vi "weight_experimental6.vi"(7 "Stop read":bool, 9 "weight source":bool, 10 "Tick":u32=100, 11 "PV weight":dbl caption="g" format="%#.0f") -> (0 "Vibration":bool caption="Вибрация", 1 "Q 2":dbl caption="mg/s" format="%#.0f", 2 "Q 1":dbl caption="mg/s" format="%#.0f", 3 "Weight 1":dbl caption="g" format="%#.0f", 5 "This VI":refnum<vi>)   [LabVIEW 2019]
uses:
  <vilib>/Analysis/baseanly.llb/Mean (DBL).vi
  Logik/fronts.vi
  Trigers/RS.vi
  Timer Delay/Timers.lvlib
  <vilib>/Analysis/NI_AALBase.lvlib
  Userlib.lvlib
  <vilib>/ptbypt/NI_PtbyPt.lvlib
panel:
  in  "Tab Control":T1(tab)=enum."Настр Ohaos"
  out "dM 2":dbl caption="g" format="%#.0f"
  out "dM 1":dbl caption="g" format="%#.0f"
  in  "Tare":dbl caption="g" format="%#.0f"
  in  "<0>":bool
  in  "<вес>":bool
  in  "k":dbl=1.0 caption="g" format="%#.3f"
  in  "Вес":dbl caption="g" format="%#.0f"
  in  "Период оценки скорости, с":i32=30
  in  "Период оценки вибрации, с":i32=20
  in  "Период усреднения, с":i32=150
  in  "Вырезать после сработки, с":i32=12
  in  "порог":dbl=480.0
  in  "Период усреднения 2":i32=50
  in  "Период оценки скорости OHAOS, с":i32=15
  in  "Период оценки вибрации OHAOS, с":i32=10
  in  "Период усреднения OHAOS, с":i32=120
  in  "Вырезать после сработки OHAOS, с":i32=5
  in  "порог OHAOS":dbl=240.0
  in  "Период усреднения OHAOS 2":i32=30
  # "Усреднение за период 1 (в настройках)"
  # "(расход)"
  # "Усреднение за период 2"
  # "(расход)"
  # "Вес тары\n(полностью очистить бункер от продукта\nи запомнить PV weight или ввести вручную)."
  # "Вес тары\n(ввести фактический вес без учета тары\nили ввести k вручную)"
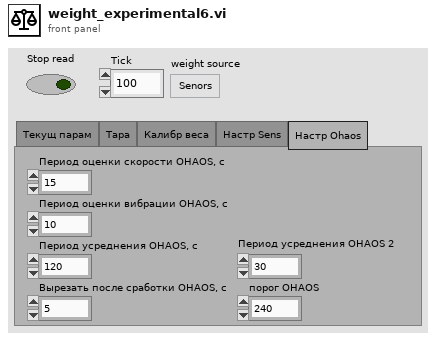
[diagram p1: front panel]
types:
  T1 = enum32{"Текущ парам", "Тара", "Калибр веса", "Настр Sens", "Настр Ohaos"}
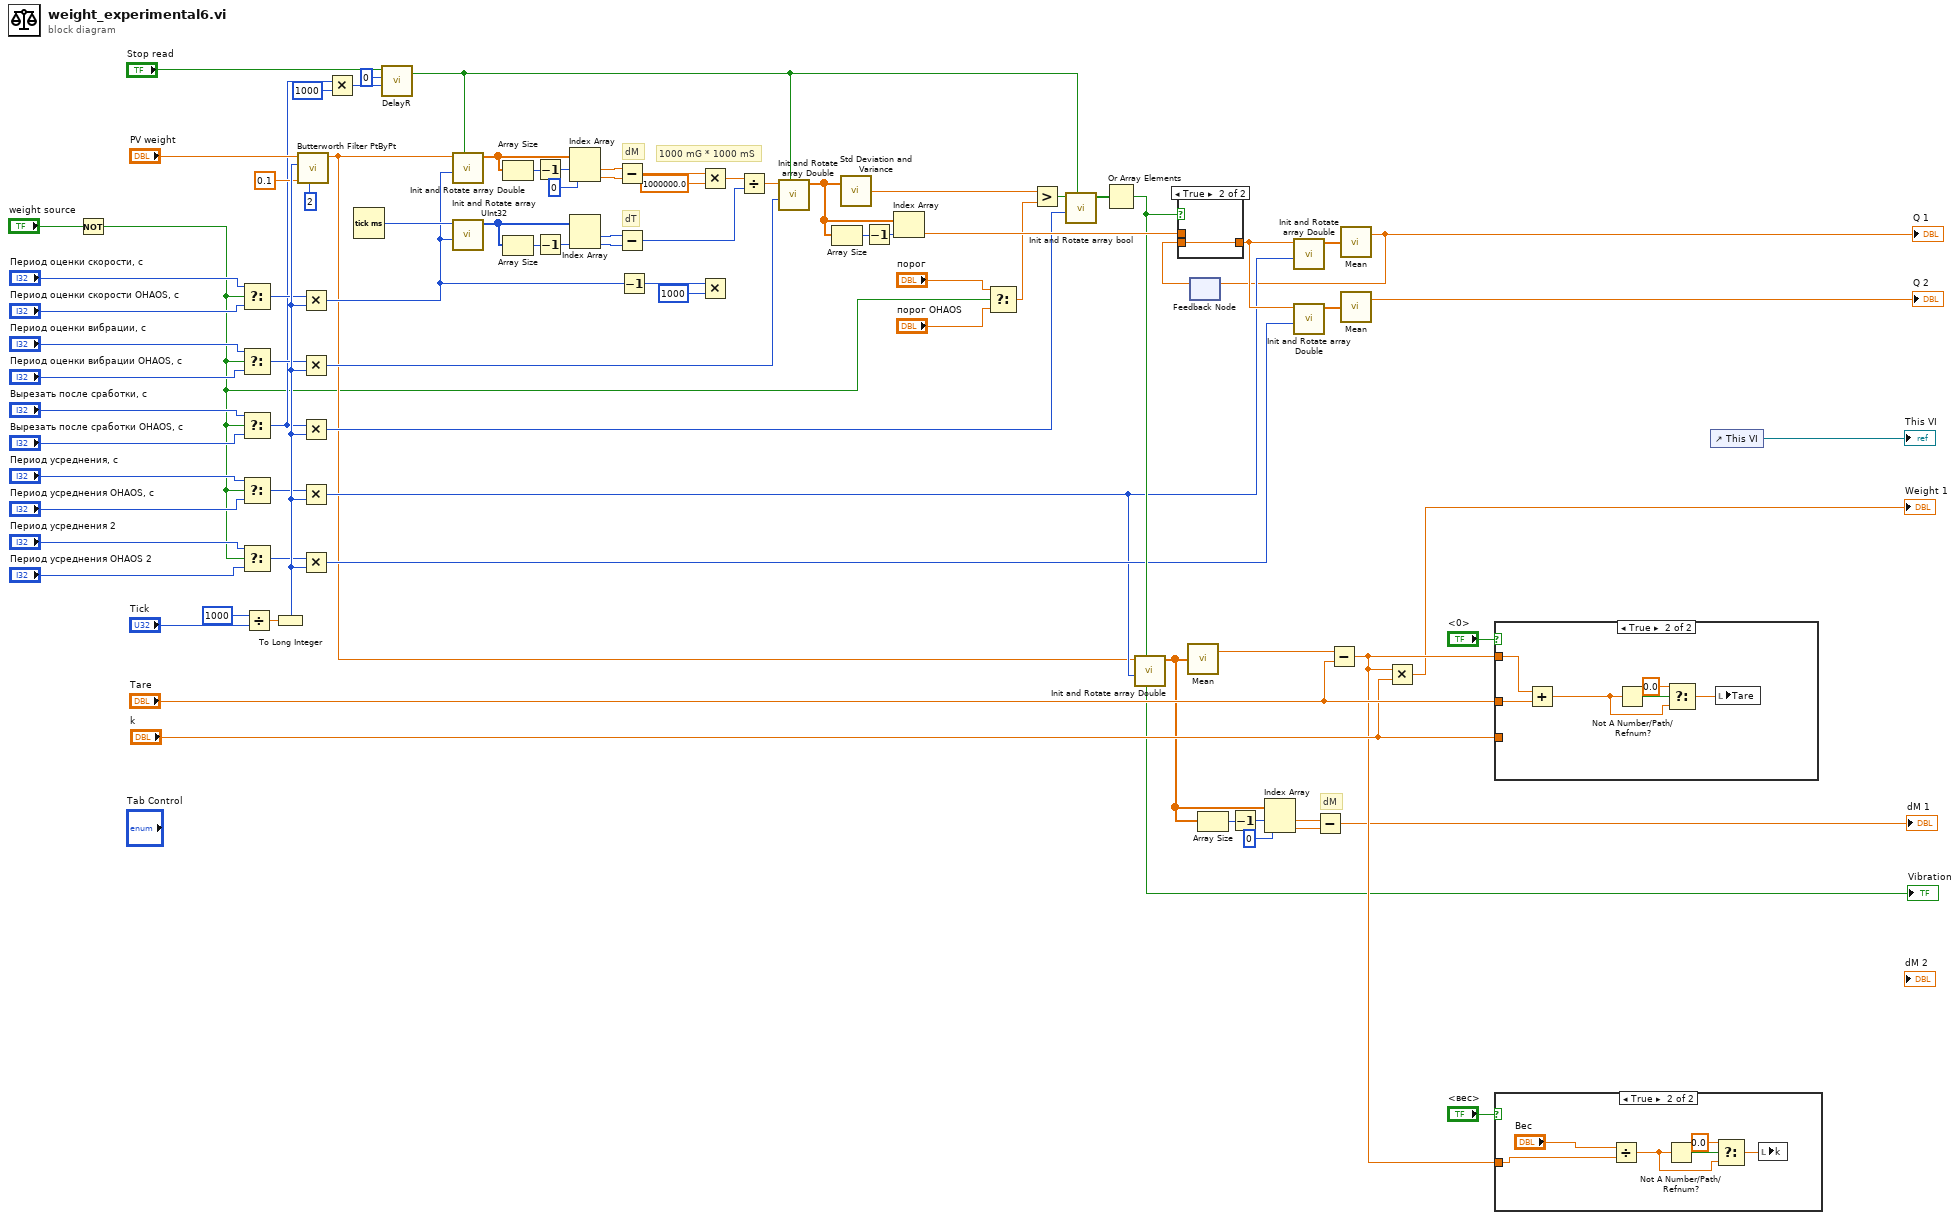
[diagram p0: block diagram]
diagram:
  # "dM"
  # "dT"
  # "1000 mG * 1000 mS"
  # "dM"
  n1 = Not(x="weight source") -> (.not. x?=w1:bool)
  n2 = Select(t="Период оценки скорости, с", s=w1, f="Период оценки скорости OHAOS, с") -> (s? t:f=w10:i32)
  n3 = Select(t="Период оценки вибрации, с", s=w1, f="Период оценки вибрации OHAOS, с") -> (s? t:f=w8:i32)
  n4 = Select(t="Вырезать после сработки, с", s=w1, f="Вырезать после сработки OHAOS, с") -> (s? t:f=w6:i32)
  n5 = Select(t="Период усреднения, с", s=w1, f="Период усреднения OHAOS, с") -> (s? t:f=w4:i32)
  n6 = Select(t="Период усреднения 2", s=w1, f="Период усреднения OHAOS 2") -> (s? t:f=w2:i32)
  n7 = Divide(x=1000 ("y"), y="Tick") -> (x/y=w33:dbl)
  n8 = To Long Integer(number=w33) -> (32bit integer=w24:i32)
  n9 = call <vilib>:"Butterworth Filter PtByPt.vi"("order"=2, "low cutoff freq: fl"=0.1, "sampling freq: fs"=w24, "x"="PV weight") -> ("Filtered x"=w21:dbl)  [unwired: 5 in, 1 out]
  n10 = Multiply(x=w10, y=w24) -> (x*y=w27:i32)
  n11 = Multiply(x=w8, y=w24) -> (x*y=w28:i32)
  n12 = Multiply(x=w6, y=w24) -> (x*y=w32:i32)
  n13 = Multiply(x=w4, y=w24) -> (x*y=w30:i32)
  n14 = Multiply(x=w2, y=w24) -> (x*y=w31:i32)
  n15 = Multiply(x=w6, y=1000) -> (x*y=w53:i32)
  n16 = Tick Count (ms)() -> (millisecond timer value=w52:u32)
  n17 = call "DelayR.vi"("DelayOff"=w53, "DelayOn"=u32 0, "In"="Stop read") -> ("Out"=w46:bool)  [unwired: 1 in, 1 out]
  n18 = call "Init and Rotate array Double.vi"("Stop read"=w46, "Array size"=w27, "PV"=w21) -> ("Array"=w73:dbl[])  [unwired: 8 in]
  n19 = call "Init and Rotate array UInt32.vi"("Array size"=w27, "PV"=w52) -> ("Array"=w50:u32[])  [unwired: 9 in]
  n20 = Array Size(array=w73) -> (size(s)=w72:i32)
  n21 = Array Size(array=w50) -> (size(s)=w51:i32)
  n22 = Decrement(x=w72) -> (x-1=w69:i32)
  n23 = Decrement(x=w51) -> (x-1=w29:i32)
  n24 = Index Array(array=w73, index #1=w69, index #2=0 ("index")) -> (element #1=w71:dbl, element #2=w70:dbl)
  n25 = Index Array(array=w50, index #2=w29) -> (element #1=w49:u32, element #2=w48:u32)  [unwired: 1 in]
  n26 = Subtract(x=w71, y=w70) -> (x-y=w77:dbl)
  n27 = Subtract(x=w49, y=w48) -> (x-y=w47:u32)
  n28 = Decrement(x=w27) -> (x-1=w64:i32)
  n29 = Multiply(x=w77, y=1000000.0) -> (x*y=w75:dbl)
  n30 = Multiply(x=w64, y=1000) -> ()  [unwired: 1 out]
  n31 = Divide(x=w75, y=w47) -> (x/y=w62:dbl)
  n32 = call "Init and Rotate array Double.vi"("Stop read"=w46, "Array size"=w28, "PV"=w62) -> ("Array"=w61:dbl[])  [unwired: 8 in]
  n33 = Array Size(array=w61) -> (size(s)=w67:i32)
  n34 = call <vilib>:"Std Deviation and Variance.vi"("X"=w61) -> ("standard deviation"=w63:dbl)  [unwired: 1 in, 2 out]
  n35 = Decrement(x=w67) -> (x-1=w66:i32)
  n36 = Index Array(array=w61, index=w66) -> (element=w65:dbl)
  n37 = Select(t="порог", s=w1, f="порог OHAOS") -> (s? t:f=w18:dbl)
  n38 = Greater?(x=w63, y=w18) -> (0:w60:bool)
  n39 = call "Init and Rotate array bool.vi"("Stop read"=w46, "Array size"=w32, "In"=w60) -> ("Array"=w59:bool[])  [unwired: 8 in]
  n40 = Or Array Elements(Boolean array=w59) -> (logical OR=w45:bool)
  "Vibration" <- w45
  n41 = call "Init and Rotate array Double.vi"("Stop read"=w45, "Array size"=w30, "PV"=w21) -> ("Array"=w40:dbl[])  [unwired: 8 in]
  n42 = call-poly <vilib>:"Mean.vi"("X"=w40) -> ("mean"=w44:dbl)  [unwired: 1 out]
  n43 = feedback #1() -> (w55:dbl)  [unwired: 1 in]
  n44 = case shown="True" w45 {
    tunnel: w55 -> [_ w88]
    tunnel: w65 -> [w87 _]
    tunnel: [w87 w88] -> w56
    frame False {
    }
    frame True {
    }
  }
  n45 = Array Size(array=w40) -> (size(s)=w43:i32)
  n46 = Decrement(x=w43) -> (x-1=w42:i32)
  n47 = Index Array(array=w40, index #1=w42, index #2=0 ("index")) -> (element #1=w39:dbl, element #2=w38:dbl)
  n48 = call "Init and Rotate array Double.vi"("Array size"=w30, "PV"=w56) -> ("Array"=w58:dbl[])  [unwired: 9 in]
  n49 = call "Init and Rotate array Double.vi"("Array size"=w31, "PV"=w56) -> ("Array"=w57:dbl[])  [unwired: 9 in]
  n50 = Subtract(x=w39, y=w38) -> (x-y=→"dM 1":dbl)
  n51 = Subtract(x=w44, y="Tare") -> (x-y=w81:dbl)
  n52 = call-poly <vilib>:"Mean.vi"("X"=w58) -> ("mean"=w26:dbl)  [unwired: 1 out]
  "Q 1" <- w26
  n53 = feedback-in #1(w26) -> ()
  n54 = call-poly <vilib>:"Mean.vi"("X"=w57) -> ("mean"=→"Q 2":dbl)  [unwired: 1 out]
  n55 = Multiply(x=w81, y="k") -> (x*y=→"Weight 1":dbl)
  n56 = case shown="True" "<0>" {
    tunnel: "Tare" -> [_ w91]
    tunnel: w81 -> [_ w90]
    tunnel: "k" -> [_ _]
    frame False {
    }
    frame True {
      n57 = Add(x=w90, y=w91) -> (x+y=w89:dbl)
      n58 = Not A Number/Path/Refnum?(number/path/refnum=w89) -> (NaN/Path/Refnum?=w94:bool)
      n59 = Select(t=0.0 ("y"), s=w94, f=w89) -> (s? t:f=w92:dbl)
      n60 = local write "Tare"(w92) -> ()
    }
  }
  n61 = case shown="True" "<вес>" {
    tunnel: w81 -> [_ w95]
    frame False {
    }
    frame True {
      n62 = Divide(x="Вес", y=w95) -> (x/y=w98:dbl)
      n63 = Not A Number/Path/Refnum?(number/path/refnum=w98) -> (NaN/Path/Refnum?=w100:bool)
      n64 = Select(t=0.0 ("y"), s=w100, f=w98) -> (s? t:f=w97:dbl)
      n65 = local write "k"(w97) -> ()
    }
  }
  n66 = control-ref of="This VI"() -> (→"This VI":refnum<vi>)
